vi "CheckOldFiles.vi"(8 "error in (no error)":errorcluster, 11 "LogFolder":path) -> (0 "error out":errorcluster)   [LabVIEW 2018]
doc: "1. Looks for existing files with _draft1 and _draft2 suffixes.\n2. Tries to open _draft1. If draft1 opens, rename to _verified and delete draft2.\n3. If draft1 fails, try to open draft2. If draft2 opens, rename to _verified and delete draft1.\n4. If draft2 fails, rename both to _failed1 and _failed2."
uses:
  <vilib>/addons/h5labview2/file/H5F.lvlib
panel:
  out "SynthesizedStrings":string[](array[string])
  out "Strings1":string[](array[string])
  out "Array":i32[](array[numeric])
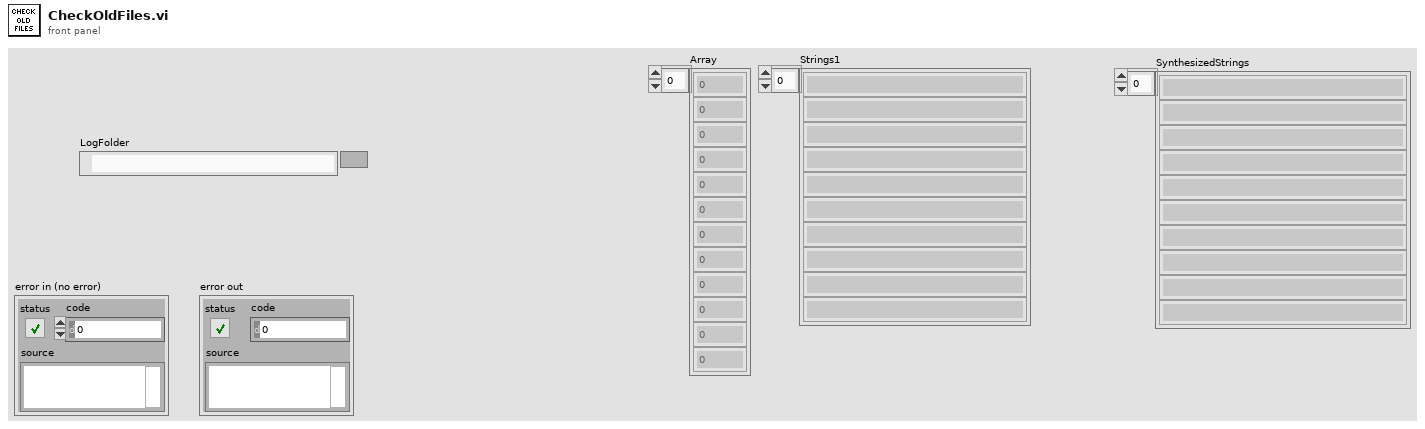
[diagram p1: front panel]
types:
  T1 = typedef "hid_t.ctl" = i32
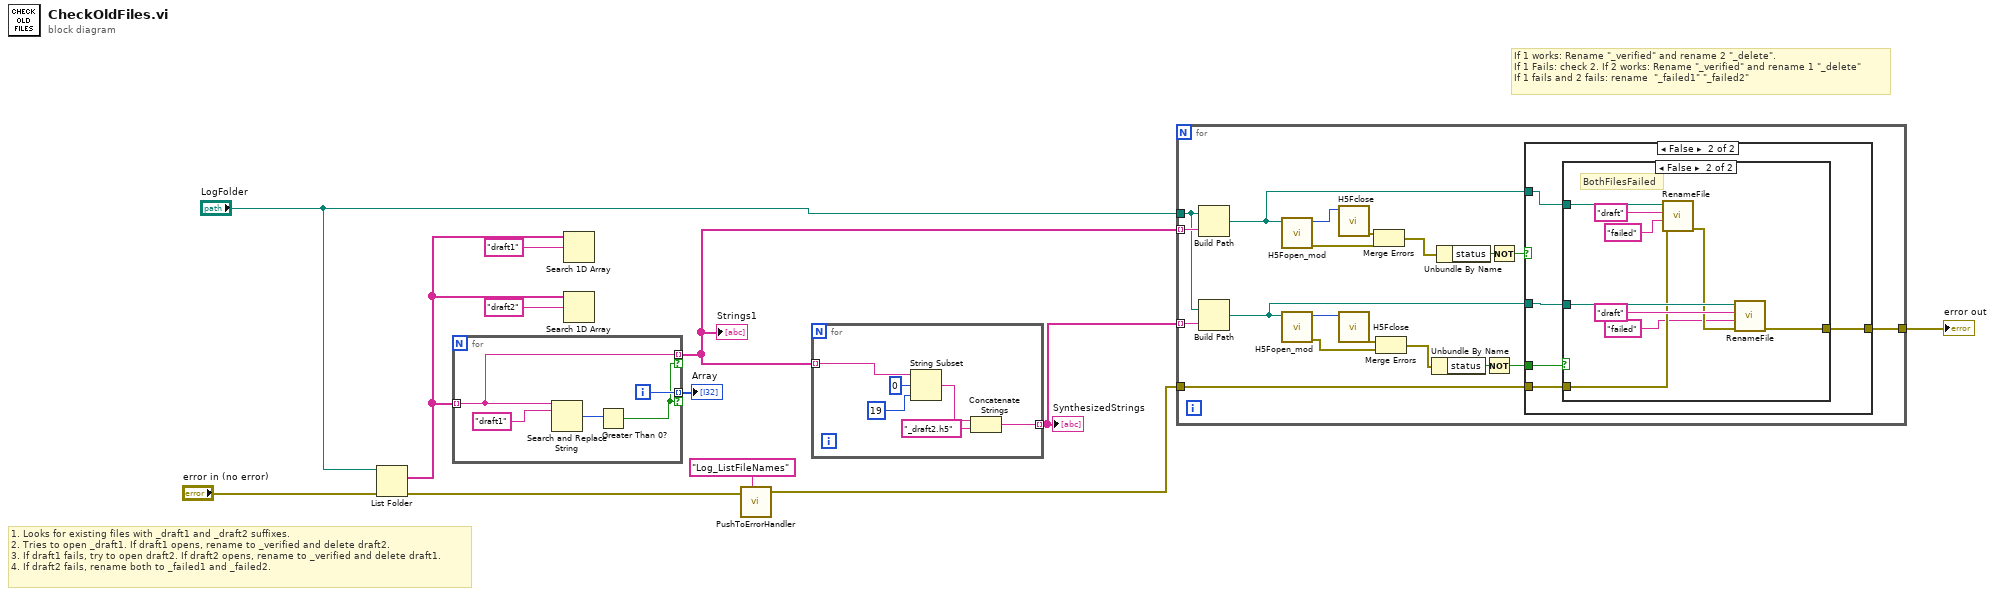
[diagram p0: block diagram]
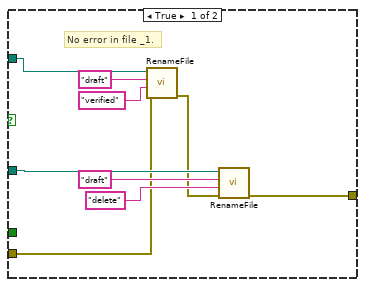
[diagram p2: hidden frame]
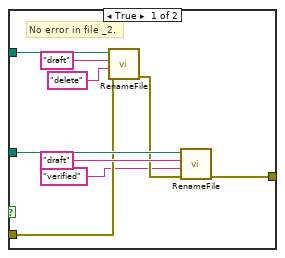
[diagram p3: hidden frame]
diagram:
  # "If 1 works: Rename \"_verified\" and rename 2 \"_delete\".\nIf 1 Fails: check 2. If 2 works: Rename \"_verified\" and rename 1 \"_delete\"\nIf 1 fails and 2 fails: rename  \"_failed1\" \"_failed2\""
  # "1. Looks for existing files with _draft1 and _draft2 suffixes.\n2. Tries to open _draft1. If draft1 opens, rename to _verified and delete draft2.\n3. If draft1 fails, try to open draft2. If draft2 opens, rename to _verified and delete draft1.\n4. If draft2 fails, rename both to _failed1 and _failed2."
  n1 = List Folder(path="LogFolder", error in="error in (no error)") -> (filenames=w9:string[], error out=w3:errorcluster)  [unwired: 2 in, 2 out]
  n2 = for {
    tunnel: w9 -> [w13] mode=indexing
    tunnel: [w15] -> w8 mode=indexing if=w14
    tunnel: [w13] -> w6 mode=indexing if=w14
    i -> [w15]
    n3 = Search and Replace String(input string=w13, search string="draft1" ("element")) -> (number of replacements=w16:i32)  [unwired: 6 in, 3 out]
    n4 = Greater Than 0?(x=w16) -> (x > 0?=w14:bool)
  }
  "Array" <- w8
  "Strings1" <- w6
  n5 = Search 1D Array(1D array=w9, element="draft1") -> ()  [unwired: 1 in, 1 out]
  n6 = Search 1D Array(1D array=w9, element="draft2") -> ()  [unwired: 1 in, 1 out]
  n7 = call "PushToErrorHandler.vi"("ErrorIn"=w3, "ErrorLocation"="Log_ListFileNames") -> ("ErrorOut"=w2:errorcluster)  [unwired: 5 in]
  n8 = for {
    tunnel: w6 -> [w23] mode=indexing
    tunnel: [w22] -> w5 mode=indexing
    n9 = String Subset(string=w23, offset (0)=0, length (rest)=19 ("length (rest)")) -> (substring=w19:string)
    n10 = Concatenate Strings(w19, "_draft2.h5" ("string")) -> (w22:string)
  }
  "SynthesizedStrings" <- w5
  n11 = for {
    tunnel: "LogFolder" -> [w40]
    tunnel: w6 -> [w42] mode=indexing
    tunnel: w5 -> [w41] mode=indexing
    tunnel: [w25] -> w1
    tunnel: w2 -> [w24]
    n12 = Build Path(base path=w40, name or relative path=w42) -> (appended path=w34:path)
    n13 = Build Path(base path=w40, name or relative path=w41) -> (appended path=w35:path)
    n14 = call "H5Fopen_mod.vi"("path"=w34) -> ("error out"=w30:errorcluster, "ref out"=w33:T1)  [unwired: 8 in, 1 out]
    n15 = call "H5Fopen_mod.vi"("path"=w35) -> ("error out"=w27:errorcluster, "ref out"=w32:T1)  [unwired: 8 in, 1 out]
    n16 = call <vilib>:"H5Fclose.vi"("ref"=w33) -> ("error out"=w31:errorcluster)  [unwired: 10 in]
    n17 = call <vilib>:"H5Fclose.vi"("ref"=w32) -> ("error out"=w28:errorcluster)  [unwired: 10 in]
    n18 = Merge Errors(w31, w30) -> (w29:errorcluster)
    n19 = Merge Errors(w28, w27) -> (w26:errorcluster)
    n20 = Unbundle By Name(w26) -> ("status"=w38:bool)
    n21 = Unbundle By Name(w29) -> ("status"=w39:bool)
    n22 = Not(x=w38) -> (.not. x?=w36:bool)
    n23 = Not(x=w39) -> (.not. x?=w37:bool)
    n24 = case shown="False" w37 {
      tunnel: w36 -> [_ w52]
      tunnel: w35 -> [w46 w55]
      tunnel: w34 -> [w51 w56]
      tunnel: [w44 w54] -> w25
      tunnel: w24 -> [w43 w53]
      frame True {
        # "No error in file _1."
        n25 = call "RenameFile.vi"("error in"=w43, "replace string (\"\")"="verified" ("replace string (\"\")"), "search string"="draft", "appended path"=w51) -> ("error out"=w45:errorcluster)  [unwired: 7 in]
        n26 = call "RenameFile.vi"("error in"=w45, "replace string (\"\")"="delete" ("replace string (\"\")"), "search string"="draft", "appended path"=w46) -> ("error out"=w44:errorcluster)  [unwired: 7 in]
      }
      frame False {
        n27 = case shown="False" w52 {
          tunnel: w56 -> [w65 w74]
          tunnel: w55 -> [w62 w71]
          tunnel: [w60 w69] -> w54
          tunnel: w53 -> [w59 w68]
          frame True {
            # "No error in file _2."
            n28 = call "RenameFile.vi"("error in"=w59, "replace string (\"\")"="delete" ("replace string (\"\")"), "search string"="draft", "appended path"=w65) -> ("error out"=w61:errorcluster)  [unwired: 7 in]
            n29 = call "RenameFile.vi"("error in"=w61, "replace string (\"\")"="verified" ("replace string (\"\")"), "search string"="draft", "appended path"=w62) -> ("error out"=w60:errorcluster)  [unwired: 7 in]
          }
          frame False {
            # "BothFilesFailed"
            n30 = call "RenameFile.vi"("error in"=w68, "replace string (\"\")"="failed" ("replace string (\"\")"), "search string"="draft", "appended path"=w74) -> ("error out"=w70:errorcluster)  [unwired: 7 in]
            n31 = call "RenameFile.vi"("error in"=w70, "replace string (\"\")"="failed" ("replace string (\"\")"), "search string"="draft", "appended path"=w71) -> ("error out"=w69:errorcluster)  [unwired: 7 in]
          }
        }
      }
    }
  }
  "error out" <- w1
